vi "Receive Control Key Down Event.vi"(8 "error in (no error)":errorcluster, 10 "ControlKeyDownMsg":refnum<class "ControlKeyDownMsg.lvclass">, 11 "ValueChangeEventProducer In":refnum<class "ValueChangeEventProducer.lvclass">) -> (0 "error out":errorcluster, 3 "ValueChangeEventProducer Out":refnum<class "ValueChangeEventProducer.lvclass">)   [LabVIEW 2017, in "Integration Test Launcher.lvlib" / "TestViewables.lvlib" / "ValueChangeEventProducer.lvclass"]
doc: "<License>\nCopyright © 2020 Tymphany, LLC | All rights reserved\nwww.Tymphany.com\nHuijun <Huijun.Guo@Tymphany.com>\n</License>"
uses:
  <vilib>/gpm_packages/@cs/example/Integration Test/ValueChangeEventProducer/ValueChangeEventProducer.lvclass
  <vilib>/gpm_packages/@cs/mva-viewable/Source/ActorEvents/IEventAggregator Messages/ControlKeyDownMsg/ControlKeyDownMsg.lvclass
  <vilib>/gpm_packages/@cs/example/Integration Test/ValueChangeEventProducer/ValueChangeEventProducer.lvclass/ValueChangeEventProducer.ctl
  <vilib>/gpm_packages/@cs/mva-viewable/Source/ActorEvents/IEventAggregator Messages/ControlKeyDownMsg/ControlKeyDownMsg.lvclass/ControlKeyDownMsg.ctl
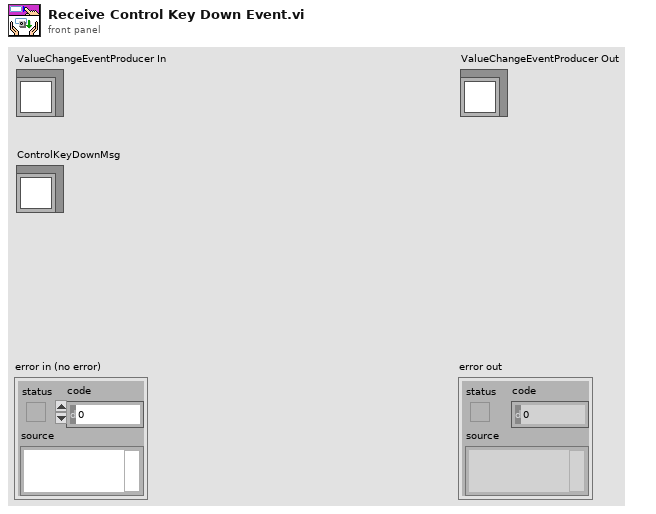
[diagram p1: front panel]
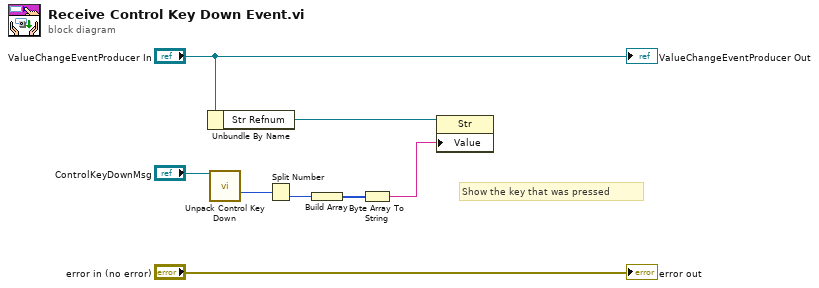
[diagram p0: block diagram]
diagram:
  # "Show the key that was pressed"
  n1 = Unbundle By Name("ValueChangeEventProducer In") -> ("Str Refnum"=w5:refnum<vi>)
  n2 = call <vilib>:"Unpack Control Key Down.vi"("ControlKeyDownMsg"="ControlKeyDownMsg") -> ("Char"=w4:i16)  [unwired: 6 in, 8 out]
  n3 = Split Number(x=w4) -> (lo(x)=w3:u8)  [unwired: 1 out]
  n4 = Build Array(w3) -> (w2:u8[])
  n5 = Byte Array To String(unsigned byte array=w2) -> (string=w1:string)
  n6 = property class="Str"(reference=w5, "Value"=w1) -> ()  [unwired: 1 in, 2 out]
  "error out" <- "error in (no error)"
  "ValueChangeEventProducer Out" <- "ValueChangeEventProducer In"
